vi "Convert Xnet CAN to BM Frame.vi"(8 "error in":errorcluster, 11 "CAN Raw Data":u8[](array[numeric])) -> (0 "error out":errorcluster, 3 "BM Frame Out":T1[](array[typedef]) {"FlexRay"."cycle count" max=63 step=1; "payload" format="%x"; "identifier / slot" format="%x"})   [LabVIEW 2014, in "CAN Bus Monitor Engine.lvlib"]
uses:
  CAN Bus Monitor Engine.lvlib
  Controls/XNET BM Frame.ctl
panel:
  in  "BM Frame":T1[](array[typedef]) {"FlexRay"."cycle count" max=63 step=1; "payload" format="%x"; "identifier / slot" format="%x"}
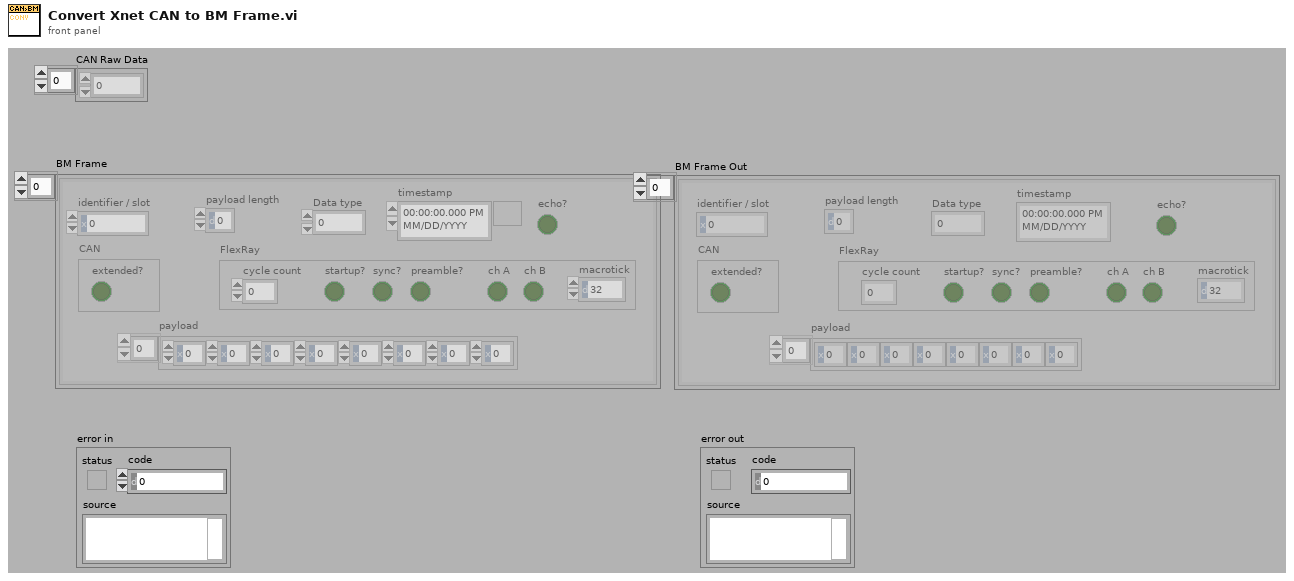
[diagram p1: front panel]
types:
  T1 = typedef "CAN Bus Monitor Engine.lvlib/XNET BM Frame.ctl" = cluster{"timestamp":timestamp, "payload":u8[], "identifier / slot":u32, "Data type":u8, "payload length":u8, "CAN":cluster{"extended?":bool}, "FlexRay":cluster{"cycle count":u8, "startup?":bool, "sync?":bool, "preamble?":bool, "ch A":bool, "ch B":bool, "macrotick":u16}, "echo?":bool}
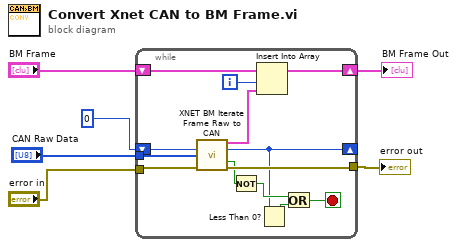
[diagram p0: block diagram]
diagram:
  n1 = while {
    tunnel: "error in" -> [w19]
    tunnel: [w18] -> w5
    tunnel: "CAN Raw Data" -> [w17]
    shift-right: [w11] -> _
    shift-left: 0 ("index out") -> [w16]
    shift-right: [w8] -> w1
    shift-left: "BM Frame" -> [w9]
    i -> [w10]
    stop <- w13 stop-if-true
    n2 = call "XNET BM Iterate Frame Raw to CAN.vi"("index in"=w16, "raw frames"=w17, "error in"=w19) -> ("output BM Frame"=w7:T1, "index out"=w11:i32, "valid?"=w15:bool, "error out"=w18:errorcluster)  [unwired: 9 in]
    n3 = Not(x=w15) -> (.not. x?=w14:bool)
    n4 = Insert Into Array(array=w9, index=w10, new element=w7) -> (w8:T1[])
    n5 = Less Than 0?(x=w11) -> (x < 0?=w12:bool)
    n6 = Or(x=w14, y=w12) -> (x .or. y?=w13:bool)
  }
  "BM Frame Out" <- w1
  "error out" <- w5
